vi "M08 TV 1.vi"(11 "NXT/EV3":T1) -> (3 "EV3 out":T1)   [LabVIEW 2016]
uses:
  <vilib>/NXT/Subs/LVHSConnector.ctl
  <vilib>/NXT/LegoClasses/BrickReference/BrickReference.lvclass
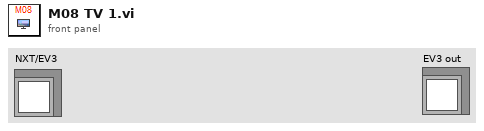
[diagram p1: front panel]
types:
  T1 = typedef "LVHSConnector.ctl" = refnum<class "BrickReference.lvclass">
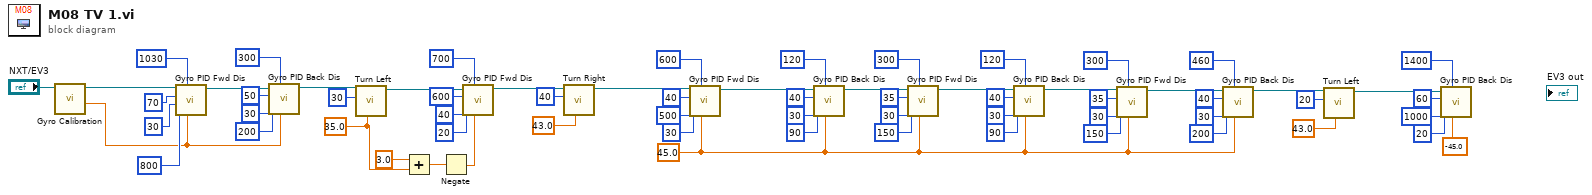
[diagram p0: block diagram]
diagram:
  w9 = sgl 45.0 ("Target angle")
  w47 = sgl 35.0 ("Turning angle")
  n1 = call "Gyro Calibration.vi"("NXT/EV3"="NXT/EV3") -> ("Degrees"=w55:sgl, "NXT/EV3"=w66:T1)  [unwired: 6 in, 1 out]
  n2 = call "Gyro PID Fwd Dis.vi"("Target angle"=w55, "Threshold to stop"=1030, "Threshold to slow"=800, "Min. speed"=30, "Max. speed"=70, "EV3 in"=w66) -> ("EV3 out"=w60:T1)  [unwired: 5 in]
  n3 = call "Gyro PID Back Dis.vi"("Target angle"=w55, "Threshold to stop"=300, "Threshold to slow"=200, "Min. speed"=30, "Max. speed"=50, "EV3 in"=w60) -> ("EV3 out"=w54:T1)  [unwired: 5 in]
  n4 = call "Turn Left.vi"("Turning angle"=w47, "Motor B (right)"=i8 30, "EV3 in"=w54) -> ("EV3 out"=w52:T1)  [unwired: 8 in]
  n5 = Add(x=sgl 3.0, y=w47) -> (x+y=w45:sgl)
  n6 = Negate(x=w45) -> (-x=w44:sgl)
  n7 = call "Gyro PID Fwd Dis.vi"("Target angle"=w44, "Threshold to stop"=700, "Threshold to slow"=20, "Min. speed"=40, "Max. speed"=600, "EV3 in"=w52) -> ("EV3 out"=w43:T1)  [unwired: 5 in]
  n8 = call "Turn Right.vi"("Turning angle"=sgl 43.0, "Motor B (right)"=i8 40, "EV3 in"=w43) -> ("EV3 out"=w40:T1)  [unwired: 8 in]
  n9 = call "Gyro PID Fwd Dis.vi"("Target angle"=w9, "Threshold to stop"=600, "Threshold to slow"=30, "Min. speed"=500, "Max. speed"=40, "EV3 in"=w40) -> ("EV3 out"=w35:T1)  [unwired: 5 in]
  n10 = call "Gyro PID Back Dis.vi"("Target angle"=w9, "Threshold to stop"=120, "Threshold to slow"=90, "Min. speed"=30, "Max. speed"=40, "EV3 in"=w35) -> ("EV3 out"=w30:T1)  [unwired: 5 in]
  n11 = call "Gyro PID Fwd Dis.vi"("Target angle"=w9, "Threshold to stop"=300, "Threshold to slow"=150, "Min. speed"=30, "Max. speed"=35, "EV3 in"=w30) -> ("EV3 out"=w25:T1)  [unwired: 5 in]
  n12 = call "Gyro PID Back Dis.vi"("Target angle"=w9, "Threshold to stop"=120, "Threshold to slow"=90, "Min. speed"=30, "Max. speed"=40, "EV3 in"=w25) -> ("EV3 out"=w19:T1)  [unwired: 5 in]
  n13 = call "Gyro PID Fwd Dis.vi"("Target angle"=w9, "Threshold to stop"=300, "Threshold to slow"=150, "Min. speed"=30, "Max. speed"=35, "EV3 in"=w19) -> ("EV3 out"=w15:T1)  [unwired: 5 in]
  n14 = call "Gyro PID Back Dis.vi"("Target angle"=w9, "Threshold to stop"=460, "Threshold to slow"=200, "Min. speed"=30, "Max. speed"=40, "EV3 in"=w15) -> ("EV3 out"=w10:T1)  [unwired: 5 in]
  n15 = call "Turn Left.vi"("Turning angle"=sgl 43.0, "Motor B (right)"=i8 20, "EV3 in"=w10) -> ("EV3 out"=w6:T1)  [unwired: 8 in]
  n16 = call "Gyro PID Back Dis.vi"("Target angle"=sgl -45.0, "Threshold to stop"=1400, "Threshold to slow"=20, "Min. speed"=1000, "Max. speed"=60, "EV3 in"=w6) -> ()  [unwired: 5 in, 1 out]
